vi "InitRW.vi"(8 "error in (no error)":errorcluster, 9 "Camera Controller":enum16{"None", "Spherical", "Flying"}(ring), 10 "Window State":T1(ring)) -> (0 "error out":errorcluster, 3 "Render Window out":refnum<class "Render Window.lvclass">)   [LabVIEW 2015, in "Render Window.lvclass"]
uses:
  Render Window.lvclass
  Render Window.lvclass/Render Window.ctl
  <vilib>/picture/3D Picture Control/NI_3D Picture Control.lvlib
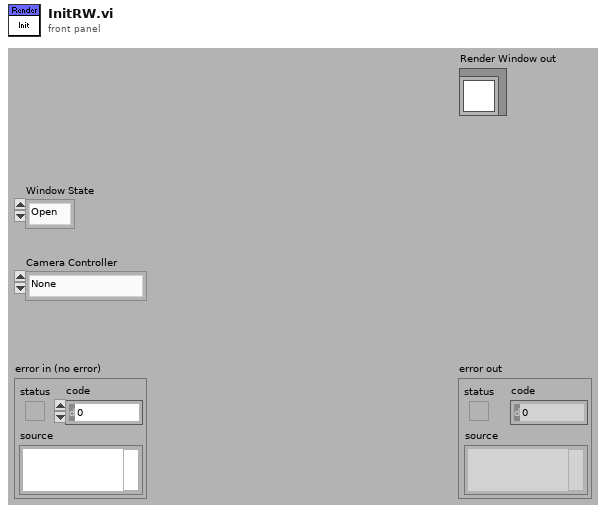
[diagram p1: front panel]
types:
  T1 = enum16{"Open", "Minimized", "Maximized", "Hidden"}
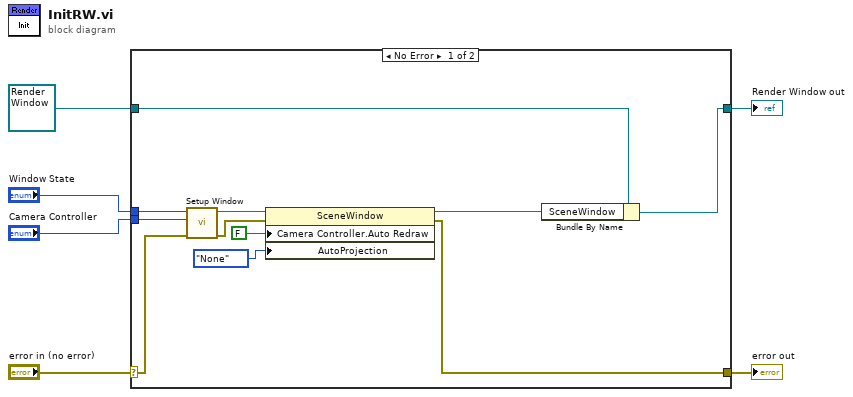
[diagram p0: block diagram]
diagram:
  n1 = case shown="No Error" "error in (no error)" {
    selector: "error in (no error)" -> [w15 w19]
    tunnel: [w9 w19] -> w5
    tunnel: [w13 w18] -> w3
    tunnel: refnum<class "Render Window.lvclass"> refnum ("Render Window in") -> [w14 w18]
    tunnel: "Window State" -> [w17 _]
    tunnel: "Camera Controller" -> [w16 _]
    frame No Error {
      n2 = call <vilib>:"Setup Window.vi"("error in (no error)"=w15, "Camera Controller"=w16, "Window State"=w17) -> ("error out"=w11:errorcluster, "New Window Refnum"=w12:refnum<vi>)  [unwired: 7 out]
      n3 = property class="SceneWindow"(reference=w12, error in=w11, "Camera Controller.Auto Redraw"=FALSE ("Camera Controller:Auto Redraw"), "AutoProjection"=enum16{"None", "Perspective", "Orthographic"}."None" ("Automatic Projection Mode")) -> (reference out=w10:refnum<vi>, error out=w9:errorcluster)
      n4 = Bundle By Name(cluster=w14, "SceneWindow"=w10) -> (w13:refnum<class "Render Window.lvclass">)
    }
    frame Error {
    }
  }
  "error out" <- w5
  "Render Window out" <- w3
